vi "TCP_close.vi"(11 "连接ID":refnum<k5>) -> (0 "error IO":errorcluster)   [LabVIEW 2013]
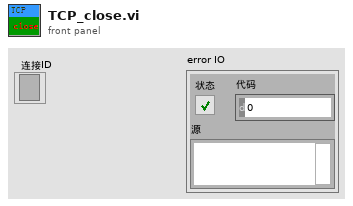
[diagram p1: front panel]
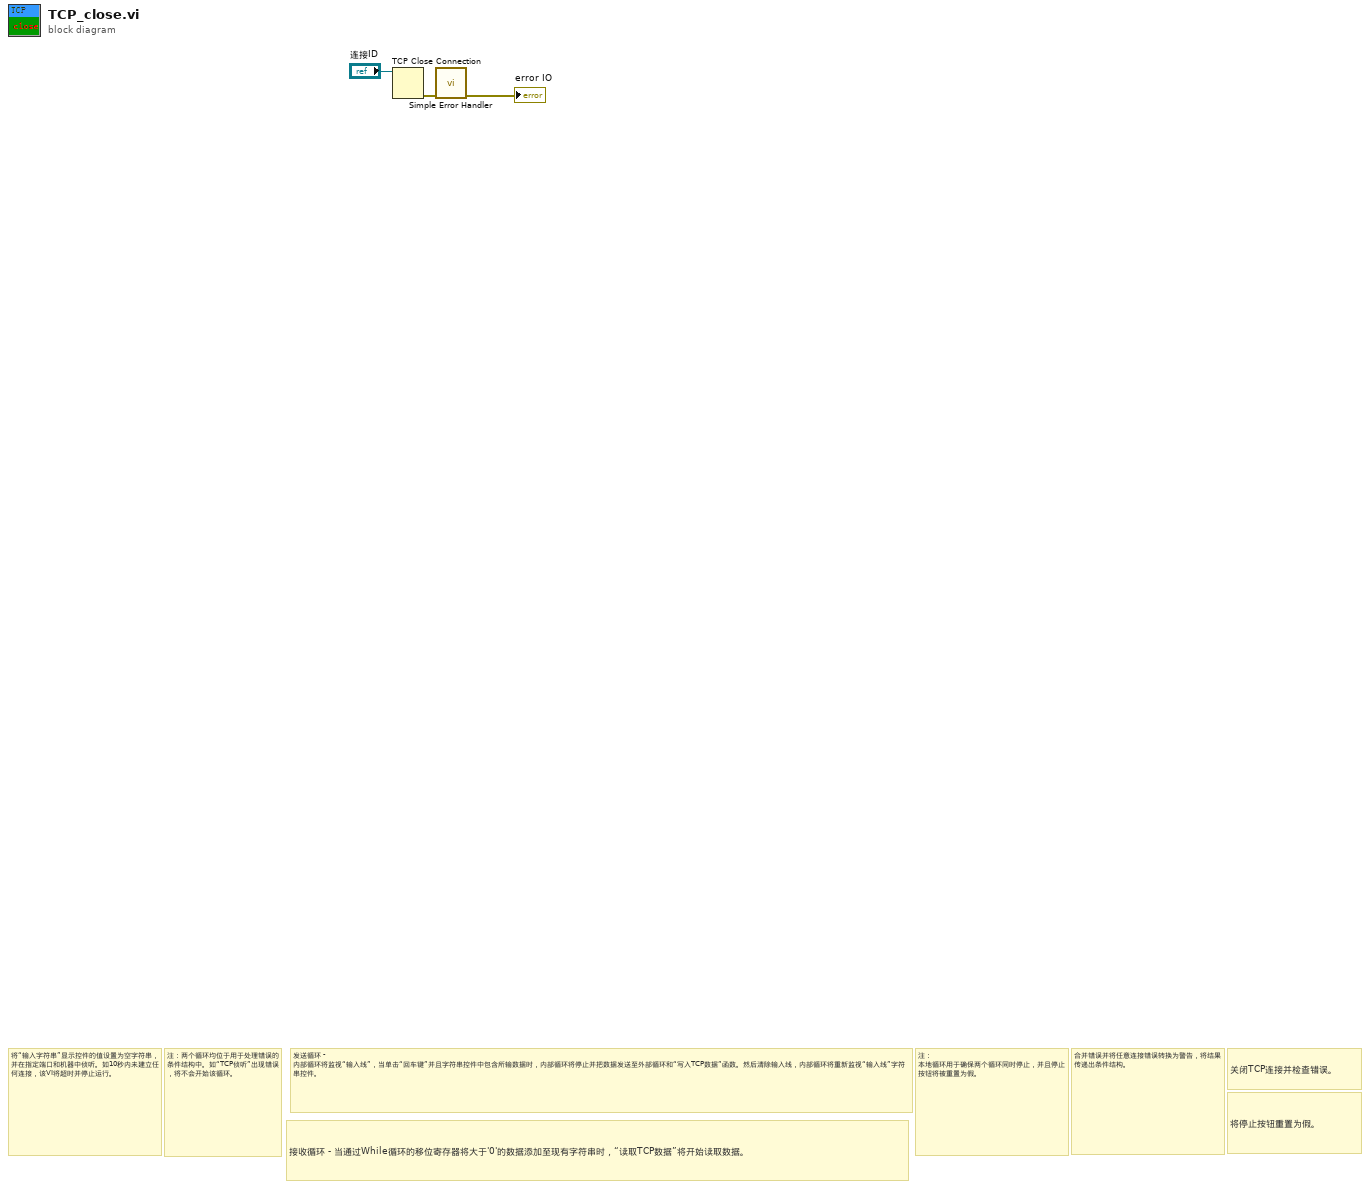
[diagram p0: block diagram]
diagram:
  # "将停止按钮重置为假。"
  # "关闭TCP连接并检查错误。"
  # "注：两个循环均位于用于处理错误的条件结构中。如“TCP侦听”出现错误，将不会开始该循环。"
  # "合并错误并将任意连接错误转换为警告，将结果传递出条件结构。"
  # "注： 本地循环用于确保两个循环同时停止，并且停止按钮将被重置为假。"
  # "接收循环 - 当通过While循环的移位寄存器将大于'0'的数据添加至现有字符串时，“读取TCP数据”将开始读取数据。"
  # "发送循环 - 内部循环将监视“输入线”，当单击“回车键”并且字符串控件中包含所输数据时，内部循环将停止并把数据发送至外部循环和“写入TCP数据”函数。然后清除输入线，内部循环将重新监视“输入线”字符串控件。"
  # "将“输入字符串”显示控件的值设置为空字符串，并在指定端口和机器中侦听。如10秒内未建立任何连接，该VI将超时并停止运行。"
  n1 = TCP Close Connection(connection ID="连接ID") -> (error out=w3:errorcluster)  [unwired: 2 in, 1 out]
  n2 = call <vilib>:"Simple Error Handler.vi"("error in (no error)"=w3) -> ("error out"=→"error IO":errorcluster)  [unwired: 4 in, 4 out]
